vi "Bias.vi"() -> ()   [LabVIEW 2016]
uses:
  controls/Enum.ctl
  <vilib>/rvi/errors/niLvFpgaAdjustHostInterfaceError.vi
  <vilib>/Utility/error.llb/Error Cluster From Error Code.vi
  controls/FPGAVIreferenceTypeDefScanEngine.ctl
  <vilib>/rvi/interface/nirviReadWriteControl/nirviReadWriteControl.xnode
  FPGA Bitfiles/qnmController797_usbRIO_controllerFPGAmu.lvbitx
  NiFpgaLv.dll
panel:
  in  "Bias (AO4)":dbl(slide) caption="Bias" scale=-10.0..10.0
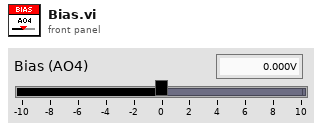
[diagram p1: front panel]
types:
  T1 = typedef "Enum.ctl" = enum16{"Init", "Read", "Write"}
  T2 = typedef "FPGAVIreferenceTypeDefScanEngine.ctl" = refnum<k20>
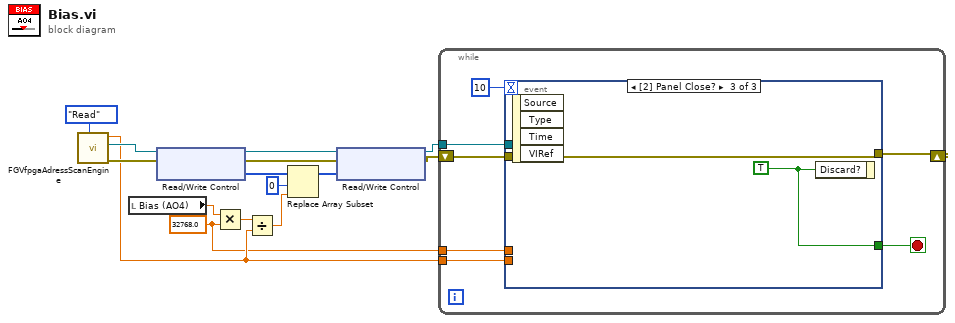
[diagram p0: block diagram]
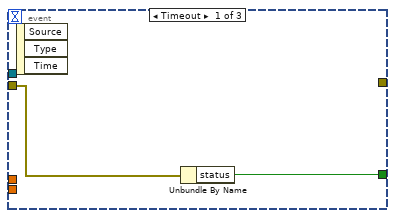
[diagram p2: hidden frame]
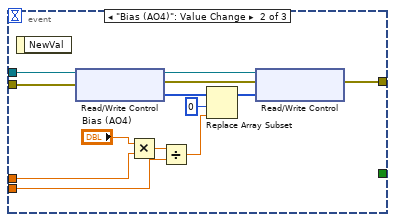
[diagram p3: hidden frame]
diagram:
  w1 = 32768.0 ("index")
  n1 = call "FGVfpgaAdressScanEngine.vi"("Enum"=Enum."Read") -> ("error out"=w6:errorcluster, "FPGA.SEout"=w15:T2, "voltageRange(+/-)Out"=w2:dbl)  [unwired: 6 in, 2 out]
  n2 = local read "Bias (AO4)"() -> (w3:dbl)
  n3 = xnode "Read/Write Control"("FPGA VI Reference In"=w15, "error in"=w6) -> ("FPGA VI Reference Out"=w7:T2, "error out"=w13:errorcluster, "aio.o.outputs"=w8:i16[])
  n4 = Multiply(x=w3, y=w1) -> (x*y=w11:dbl)
  n5 = Divide(x=w11, y=w2) -> (x/y=w12:dbl)
  n6 = Replace Array Subset(array=w8, new element=w12, index=0) -> (w9:i16[])
  n7 = xnode "Read/Write Control"("FPGA VI Reference In"=w7, "error in"=w13, "aio.o.outputs"=w9) -> ("FPGA VI Reference Out"=w4:T2, "error out"=w5:errorcluster)
  n8 = while {
    tunnel: w2 -> [w19]
    shift-right: [w18] -> _
    shift-left: w5 -> [w17]
    tunnel: w1 -> [w16]
    tunnel: w4 -> [w20]
    stop <- w22 stop-if-true
    n9 = event shown="[2] Panel Close?" {
      selector: _ -> [_ _ _]
      dyn-events: _ -> [_ _ _]
      timeout: 10 -> [_ _ _]
      tunnel: [w23 _ w39] -> w22
      tunnel: w20 -> [_ w28 _]
      tunnel: w19 -> [_ w26 _]
      tunnel: [_ w29 w38] -> w18
      tunnel: w17 -> [w24 w27 w38]
      tunnel: w16 -> [_ w25 _]
      event Timeout {
        n10 = event-data() -> ()  [unwired: 1 in, 3 out]
        n11 = Unbundle By Name(w24) -> ("status"=w23:bool)
      }
      event "Bias (AO4)": Value Change {
        n12 = event-data() -> ()  [unwired: 1 in, 1 out]
        n13 = xnode "Read/Write Control"("FPGA VI Reference In"=w28, "error in"=w27) -> ("FPGA VI Reference Out"=w37:T2, "error out"=w30:errorcluster, "aio.o.outputs"=w36:i16[])
        n14 = Multiply(x="Bias (AO4)", y=w25) -> (x*y=w32:dbl)
        n15 = Divide(x=w32, y=w26) -> (x/y=w31:dbl)
        n16 = Replace Array Subset(array=w36, new element=w31, index=0) -> (w35:i16[])
        n17 = xnode "Read/Write Control"("FPGA VI Reference In"=w37, "error in"=w30, "aio.o.outputs"=w35) -> ("error out"=w29:errorcluster)  [unwired: 1 out]
      }
      event Panel Close? {
        w39 = TRUE ("Discard?")
        n18 = event-data() -> ()  [unwired: 1 in, 4 out]
        n19 = event-data("Discard?"=w39) -> ()  [unwired: 1 in, 1 out]
      }
    }
  }
